vi "Build core.vi"(6 "Previous Build's Artifacts":refnum<class "Build Artifact.lvclass">[](array[class]), 7 "Progress":refnum<class "Progress.lvclass">, 8 "error in (no error)":errorcluster, 10 "Build Cache":refnum<class "Build Cache.lvclass">, 11 "Close VIPM Step in":refnum<class "Close VIPM Step.lvclass">) -> (0 "error out":errorcluster, 1 "Explore Path":path, 2 "Build Results":T1, 4 "New Artifacts":refnum<class "Build Artifact.lvclass">[](array[class]))   [LabVIEW 2019, in "VIPM.lvlib" / "Close VIPM Step.lvclass"]
doc: "Performs all the necessary build actions for the build step.\n\nCopyright: MGI 2016\nAuthor: Derek Trepanier"
uses:
  Close VIPM Step.lvclass
  libs/Solution.lvlibp/Solution/Progress/Progress.lvclass
  libs/Solution.lvlibp/Solution/Build Artifact/Build Artifact.lvclass
  libs/Solution.lvlibp/Solution/Build Item/Build Result.ctl
  libs/Solution.lvlibp/Solution/Build Cache/Build Cache.lvclass
  <vilib>/JKI/VIPM API/VIPM API_vipm_api.lvlib
  libs/Solution.lvlibp/Solution/Build Item/Build Step.lvclass
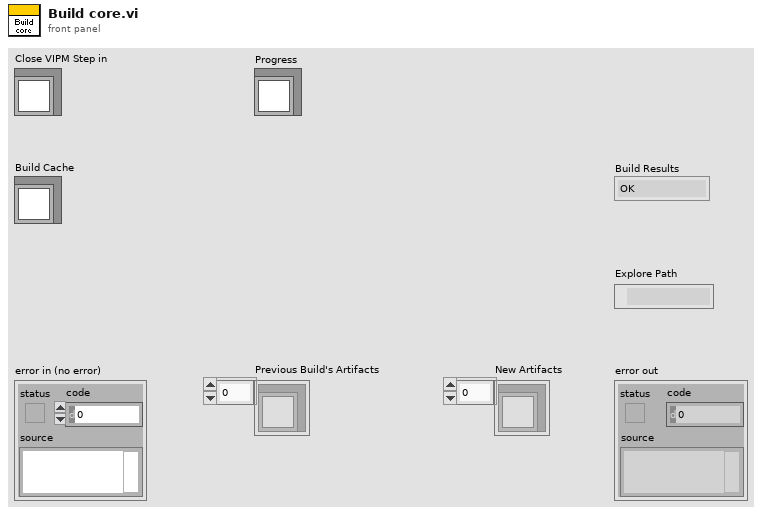
[diagram p1: front panel]
types:
  T1 = typedef "Solution.lvlibp/Build Step.lvclass/Build Result.ctl" = enum16{"OK", "Skipped", "Error"}
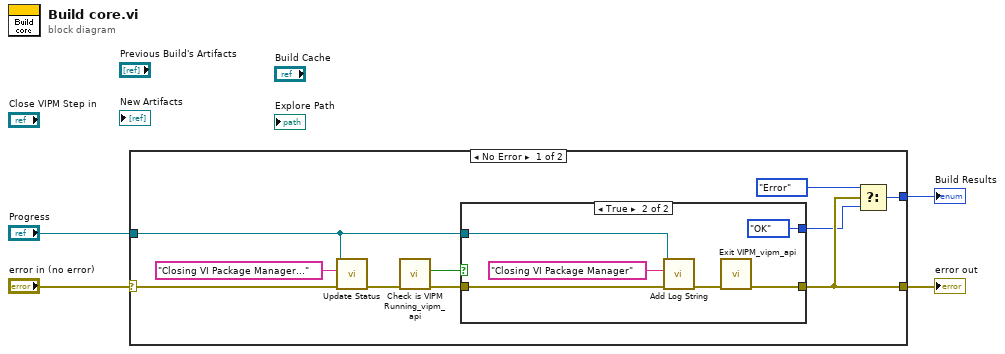
[diagram p0: block diagram]
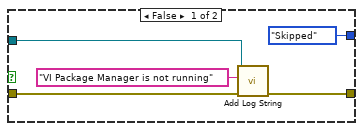
[diagram p2: hidden frame]
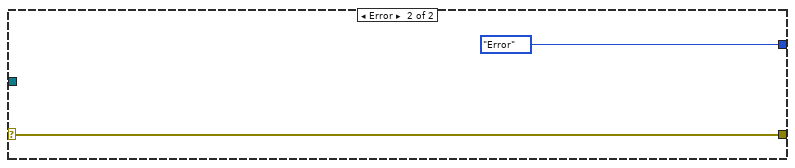
[diagram p3: hidden frame]
diagram:
  n1 = case shown="No Error" "error in (no error)" {
    selector: "error in (no error)" -> [w8 w26]
    tunnel: [w12 w26] -> w3
    tunnel: [w10 Build_Result."Error" ("Build Results")] -> w2
    tunnel: "Progress" -> [w6 _]
    frame No Error {
      n2 = call "Update Status.vi"("error in (no error)"=w8, "Status String"="Closing VI Package Manager...", "Progress in"=w6) -> ("error out"=w7:errorcluster)  [unwired: 8 in]
      n3 = call <vilib>:"Check is VIPM Running_vipm_api.vi"("error in (no error)"=w7) -> ("error out"=w14:errorcluster, "is Running"=w13:bool)  [unwired: 9 in]
      n4 = case shown="True" w13 {
        tunnel: w14 -> [w18 w24]
        tunnel: [w19 w25] -> w12
        tunnel: [Build_Result."Skipped" ("Build Results") Build_Result."OK" ("Build Results")] -> w11
        tunnel: w6 -> [w15 w20]
        frame False {
          n5 = call "Add Log String.vi"("error in (no error)"=w18, "Log Item"="VI Package Manager is not running", "Progress in"=w15) -> ("error out"=w19:errorcluster)  [unwired: 8 in]
        }
        frame True {
          n6 = call "Add Log String.vi"("error in (no error)"=w24, "Log Item"="Closing VI Package Manager", "Progress in"=w20) -> ("error out"=w23:errorcluster)  [unwired: 8 in]
          n7 = call <vilib>:"Exit VIPM_vipm_api.vi"("error in (no error)"=w23) -> ("error out"=w25:errorcluster)  [unwired: 10 in]
        }
      }
      n8 = Select(t=Build_Result."Error", s=w12, f=w11) -> (s? t:f=w10:T1)
    }
    frame Error {
    }
  }
  "error out" <- w3
  "Build Results" <- w2
